vi "Check For Pin Out Of Range.vi"(8 "Error In":errorcluster, 9 "Pin Type":T1, 10 "User Pin Number":u8, 11 "Arduino Resource":T2={"COM Port"="", "Board Type"=enum."ChipKit Uno32", "Connection Type"=enum."USB / Serial", "Baud Rate (115200)"=15, "Bytes Per Packet (15)"=15}) -> (0 "Error Out":errorcluster, 3 "Arduino Resource":T2={"COM Port"="", "Board Type"=enum."ChipKit Uno32", "Connection Type"=enum."USB / Serial", "Baud Rate (115200)"=15, "Bytes Per Packet (15)"=15})   [LabVIEW 2011, in "LabVIEW Interface for ChipKit.lvlib"]
uses:
  LabVIEW Interface for ChipKit.lvlib
  Private/Type Defs/Chipkit Resource.ctl
  Private/Type Defs/Board Type.ctl
  Private/Type Defs/Connection Type.ctl
  Private/Type Defs/Pin Type.ctl
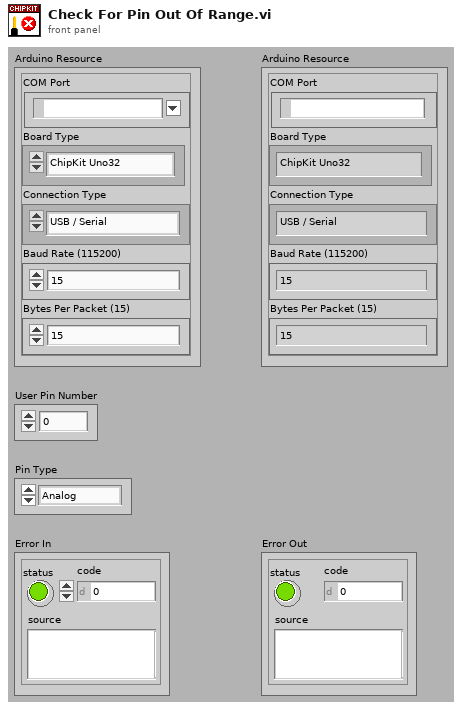
[diagram p1: front panel]
types:
  T1 = typedef "LabVIEW Interface for ChipKit.lvlib/Pin Type.ctl" = enum8{"Analog", "Digital"}
  T2 = typedef "LabVIEW Interface for ChipKit.lvlib/Chipkit Resource.ctl" = cluster{"COM Port":refnum<visa-resource-name>, "Board Type":T3, "Connection Type":T4, "Baud Rate (115200)":u32, "Bytes Per Packet (15)":u32}
  T3 = typedef "LabVIEW Interface for ChipKit.lvlib/Board Type.ctl" = enum16{"ChipKit uC32", "ChipKit Uno32", "ChipKit Max32"}
  T4 = typedef "LabVIEW Interface for ChipKit.lvlib/Connection Type.ctl" = enum8{"USB / Serial", "XBEE", "BlueSmirf (Bluetooth)"}
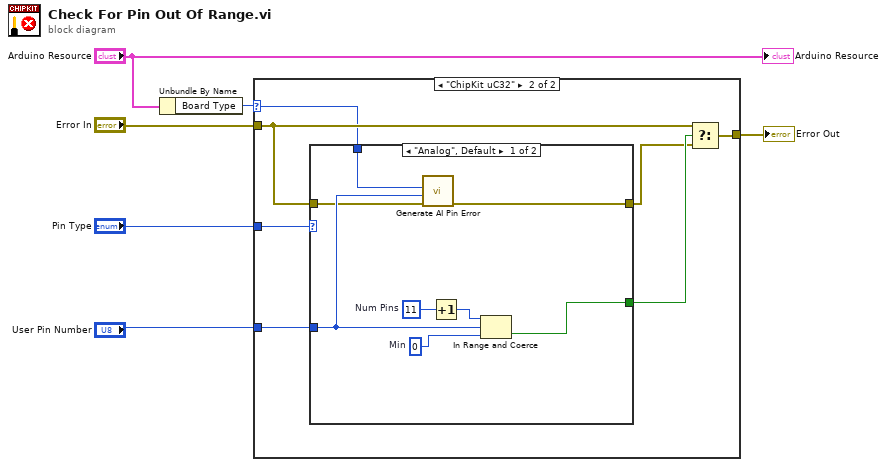
[diagram p0: block diagram]
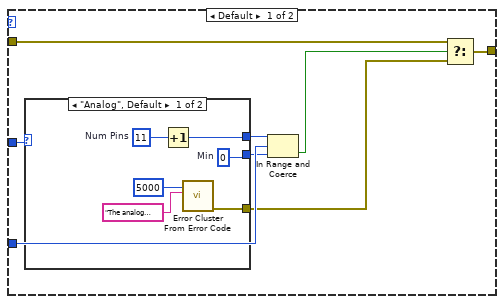
[diagram p2: hidden frame]
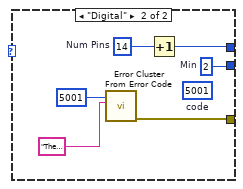
[diagram p3: hidden frame]
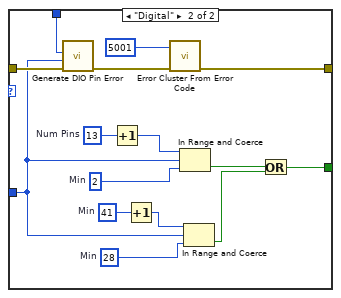
[diagram p4: hidden frame]
diagram:
  n1 = Unbundle By Name("Arduino Resource") -> ("Board Type"=w1:T3)
  n2 = case shown="\"ChipKit uC32\"" w1 {
    selector: w1 -> [_ w27]
    tunnel: "User Pin Number" -> [w13 w31]
    tunnel: "Error In" -> [w9 w28]
    tunnel: [w14 w33] -> w5
    tunnel: "Pin Type" -> [w12 w32]
    frame Default {
      n3 = case shown="\"Analog\", Default" w12 {
        tunnel: [w20 w26] -> w11
        tunnel: [w15 w21] -> w10
        tunnel: [w18 w23] -> w7
        frame "Analog", Default {
          w16 = u8 11  # Num Pins
          w20 = u8 0  # Min
          n4 = Increment(x=w16) -> (x+1=w15:u8)
          n5 = call <vilib>:"Error Cluster From Error Code.vi"("error message (\"\")"="The analog input pin selected does not exist on the specified board.  Ensure that the correct board type and analog pin values are specified." ("source"), "error code (0)"=5000) -> ("error out"=w18:errorcluster)  [unwired: 7 in]
        }
        frame "Digital" {
          (unwired) 5001  # code
          w22 = u8 14  # Num Pins
          w26 = u8 2  # Min
          n6 = call <vilib>:"Error Cluster From Error Code.vi"("error message (\"\")"="The digital input pin selected is not available on the specified board.  Ensure that the correct board type and digital pin values are specified.\nNote: Digital pins 0 and 1 are used for serial communication between LabVIEW and the ChipKit and cannot be used for digital I/O." ("source"), "error code (0)"=5001) -> ("error out"=w23:errorcluster)  [unwired: 7 in]
          n7 = Increment(x=w22) -> (x+1=w21:u8)
        }
      }
      n8 = In Range and Coerce(upper limit=w10, x=w13, lower limit=w11) -> (In Range?=w8:bool)  [unwired: 1 out]
      n9 = Select(t=w9, s=w8, f=w7) -> (s? t:f=w14:errorcluster)
    }
    frame "ChipKit uC32" {
      n10 = case shown="\"Analog\", Default" w32 {
        tunnel: [w35 w55] -> w29
        tunnel: w31 -> [w36 w42]
        tunnel: [w38 w46] -> w30
        tunnel: w28 -> [w34 w45]
        tunnel: w27 -> [w37 w43]
        frame "Analog", Default {
          w41 = u8 11  # Num Pins
          w39 = u8 0  # Min
          n11 = call "Generate AI Pin Error.vi"("Error In"=w34, "Pin Number"=w36, "Board Type"=w37) -> ("Error Out"=w35:errorcluster)  [unwired: 8 in]
          n12 = Increment(x=w41) -> (x+1=w40:u8)
          n13 = In Range and Coerce(upper limit=w40, x=w36, lower limit=w39) -> (In Range?=w38:bool)  [unwired: 1 out]
        }
        frame "Digital" {
          w51 = u8 41  # Min
          w49 = u8 28  # Min
          w54 = u8 13  # Num Pins
          w52 = u8 2  # Min
          n14 = call "Generate DIO Pin Error.vi"("Error In"=w45, "Pin Number"=w42, "Board Type"=w43) -> ("Error Out"=w44:errorcluster)  [unwired: 8 in]
          n15 = Increment(x=w54) -> (x+1=w53:u8)
          n16 = Increment(x=w51) -> (x+1=w50:u8)
          n17 = call <vilib>:"Error Cluster From Error Code.vi"("error in (no error)"=w44, "error code (0)"=5001) -> ("error out"=w55:errorcluster)  [unwired: 7 in]
          n18 = In Range and Coerce(upper limit=w53, x=w42, lower limit=w52) -> (In Range?=w48:bool)  [unwired: 1 out]
          n19 = In Range and Coerce(upper limit=w50, x=w42, lower limit=w49) -> (In Range?=w47:bool)  [unwired: 1 out]
          n20 = Or(x=w48, y=w47) -> (x .or. y?=w46:bool)
        }
      }
      n21 = Select(t=w28, s=w30, f=w29) -> (s? t:f=w33:errorcluster)
    }
  }
  "Error Out" <- w5
  "Arduino Resource" <- "Arduino Resource"
